vi "PPFS_DRIVE_MODULE_OPEN.vi"(3 "Module Index":i32, 4 "RadiansPerCount":dbl=1.0, 5 "Drive PWM Channel":T2, 6 "DistancePerCount":dbl=1.0, 7 "Swerve PWM Channel":T2, 8 "Swerve B Channel":T1, 9 "Swerver A Channel":T1, 10 "Drive B Channel":T1, 11 "Drive A channel":T1) -> ()   [LabVIEW 2019]
uses:
  <vilib>/Rock Robotics/SystemInterfaces/DIO/FPGA_DIOChannel.ctl
  <vilib>/Rock Robotics/SystemInterfaces/DIO/FPGA_DIOPWMChannel.ctl
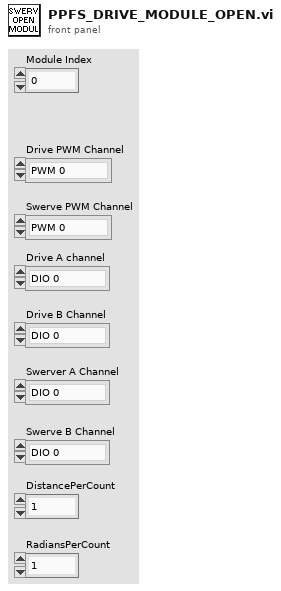
[diagram p1: front panel]
types:
  T1 = typedef "FPGA_DIOChannel.ctl" = enum8{"DIO 0", "DIO 1", "DIO 2", "DIO 3", "DIO 4", "DIO 5", "DIO 6", "DIO 7", "DIO 8", "DIO 9", "DIO MXP 0", "DIO MXP 1", "DIO MXP 2", "DIO MXP 3", "DIO MXP 4", "DIO MXP 5", "DIO MXP 6", "DIO MXP 7", "DIO MXP 8", "DIO MXP 9", "DIO MXP 10", "DIO MXP 11", "DIO MXP 12", "DIO MXP 13", "DIO MXP 14", "DIO MXP 15", "SPI Port CS1", "SPI Port CS2", "SPI Port CS3", "SPI Port MISO", "SPI Port MOSI", "Invalid"}
  T2 = typedef "FPGA_DIOPWMChannel.ctl" = enum8{"PWM 0", "PWM 1", "PWM 2", "PWM 3", "PWM 4", "PWM 5", "PWM 6", "PWM 7", "PWM 8", "PWM 9", "PWM MXP 0", "PWM MXP 1", "PWM MXP 2", "PWM MXP 3", "PWM MXP 4", "PWM MXP 5", "PWM MXP 6", "PWM MXP 7", "PWM MXP 8", "PWM MXP 9", "Invalid"}
  T3 = typedef "WPI_EncoderDevRef.ctl" = cluster{"DevStatus":errorcluster, "EncoderIndex":T4, "CounterIndex":T5, "DistancePerCount":dbl, "Decoding Type":T6}
  T4 = typedef "FPGA_EncoderIdx.ctl" = enum8{"Enc 0", "Enc 1", "Enc 2", "Enc 3", "Enc 4", "Enc 5", "Enc 6", "Enc 7", "Invalid"}
  T5 = typedef "FPGA_CounterCtrSystemIndex.ctl" = enum8{"Ctr 0", "Ctr 1", "Ctr 2", "Ctr 3", "Ctr 4", "Ctr 5", "Ctr 6", "Ctr 7", "Invalid"}
  T6 = typedef "WPI_EncoderType.ctl" = enum16{"1x", "2x", "4x"}
  T7 = typedef "WPI_MotorControlDeviceRef.ctl" = cluster{"DeviceStatus":errorcluster, "Type":T8, "PWM":cluster{"PWM Channel":T2, "DeadBand":T9}, "CAN":cluster{"Device Number":u8, "SetOutput VI Ref":variant, "GetOutput VI Ref":variant, "Enable VI Ref":variant, "Disable VI Ref":variant, "Data":variant}, "Invert":bool, "DIO PWM":cluster{"PWM \"Enable\" Channel":T2, "DIOChannel":T1, "PWM Rate":dbl}}
  T8 = typedef "WPI_MotorControlType.ctl" = enum16{"PWM", "CAN", "DIO PWM"}
  T9 = typedef "WPI_PWMDeadband.ctl" = cluster{"Name":string, "maxPositivePwm":i32, "minPositivePwm":i32, "centerPwm":i32, "maxNegativePwm":i32, "minNegativePwm":i32, "angularRange":u16}
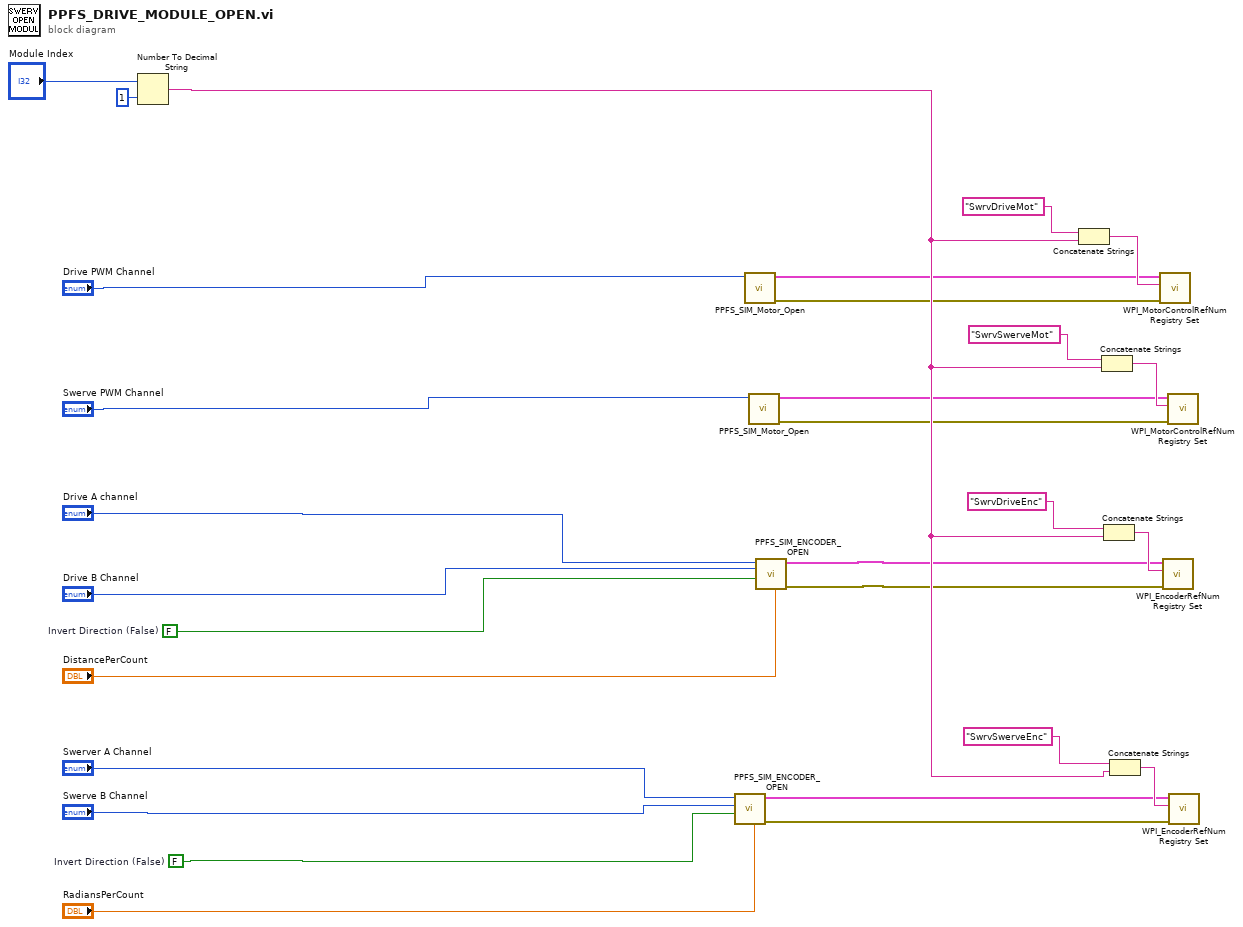
[diagram p0: block diagram]
diagram:
  w1 = FALSE  # Invert Direction (False)
  w2 = FALSE  # Invert Direction (False)
  n1 = Number To Decimal String(number="Module Index", width (-)=i16 1) -> (decimal integer string=w11:string)
  n2 = call "PPFS_SIM_ENCODER_OPEN.vi"("DistancePerCount"="RadiansPerCount", "Invert"=w2, "DIO Channel B"="Swerve B Channel", "DIO Channel  A"="Swerver A Channel") -> ("error out"=w4:errorcluster, "SwerveDriveEnc"=w3:T3)  [unwired: 6 in]
  n3 = call "PPFS_SIM_Motor_Open.vi"("PWM Channel"="Drive PWM Channel") -> ("error out"=w8:errorcluster, "Motor Device Reference"=w7:T7)  [unwired: 9 in]
  n4 = call "PPFS_SIM_Motor_Open.vi"("PWM Channel"="Swerve PWM Channel") -> ("error out"=w10:errorcluster, "Motor Device Reference"=w9:T7)  [unwired: 9 in]
  n5 = call "PPFS_SIM_ENCODER_OPEN.vi"("DistancePerCount"="DistancePerCount", "Invert"=w1, "DIO Channel B"="Drive B Channel", "DIO Channel  A"="Drive A channel") -> ("error out"=w6:errorcluster, "SwerveDriveEnc"=w5:T3)  [unwired: 6 in]
  n6 = Concatenate Strings("SwrvDriveMot" ("refnum name"), w11) -> (w12:string)
  n7 = Concatenate Strings("SwrvSwerveMot" ("refnum name"), w11) -> (w13:string)
  n8 = Concatenate Strings("SwrvDriveEnc" ("refnum name"), w11) -> (w14:string)
  n9 = Concatenate Strings("SwrvSwerveEnc" ("refnum name"), w11) -> (w15:string)
  n10 = call <vilib>:"WPI_MotorControlRefNum Registry Set.vi"("error in (no error)"=w8, "refnum name"=w12, "MotorControlDevRef"=w7) -> ()  [unwired: 7 in, 2 out]
  n11 = call <vilib>:"WPI_EncoderRefNum Registry Set.vi"("error in (no error)"=w6, "refnum name"=w14, "EncoderDevRef"=w5) -> ()  [unwired: 7 in, 2 out]
  n12 = call <vilib>:"WPI_MotorControlRefNum Registry Set.vi"("error in (no error)"=w10, "refnum name"=w13, "MotorControlDevRef"=w9) -> ()  [unwired: 7 in, 2 out]
  n13 = call <vilib>:"WPI_EncoderRefNum Registry Set.vi"("error in (no error)"=w4, "refnum name"=w15, "EncoderDevRef"=w3) -> ()  [unwired: 7 in, 2 out]
